vi "GetDisplayClick.vi"(0 "Display REFs In":refnum<vi>[](array[refnum]), 11 "Calling VI REF":refnum<vi>) -> (8 "Display Index":i32)   [LabVIEW 2014]
uses:
  <vilib>/Utility/cursorutil.llb/Set Cursor (Icon Pict).vi
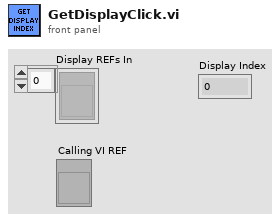
[diagram p1: front panel]
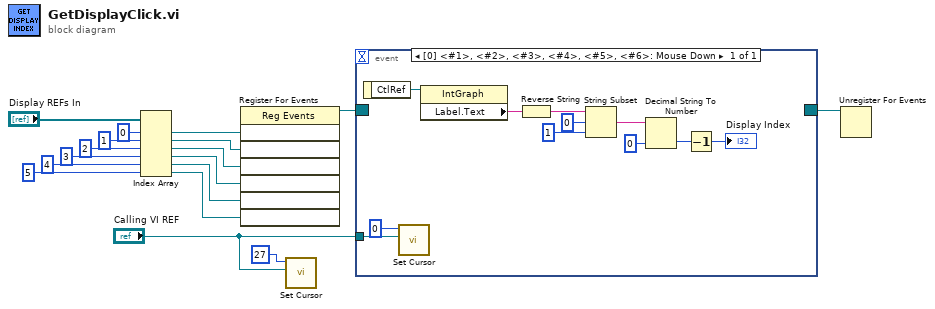
[diagram p0: block diagram]
diagram:
  n1 = Index Array(array="Display REFs In", index #1=0 ("index"), index #2=1 ("index"), index #3=2 ("index"), index #4=3 ("index"), index #5=4 ("index"), index #6=5 ("index")) -> (element #1=w4:refnum<vi>, element #2=w7:refnum<vi>, element #3=w8:refnum<vi>, element #4=w9:refnum<vi>, element #5=w10:refnum<vi>, element #6=w11:refnum<vi>)
  n2 = register-events(w4, w7, w8, w9, w10, w11) -> (reference out=w6:refnum<event-registration>)  [unwired: 2 in, 1 out]
  n3 = call-poly <vilib>:"Set Cursor.vi"("VI reference (current VI)"="Calling VI REF", "icon"=u16 27) -> ()  [unwired: 8 in, 2 out]
  n4 = event shown="[0] <#1>, <#2>, <#3>, <#4>, <#5>, <#6>: Mouse Down" {
    selector: w6 -> [_]
    dyn-events: [_] -> w5
    timeout: _ -> [_]
    tunnel: "Calling VI REF" -> [w27]
    event Mouse Down {
      n5 = event-data() -> ("CtlRef"=w26:refnum<vi>)  [unwired: 1 in]
      n6 = call-poly <vilib>:"Set Cursor.vi"("VI reference (current VI)"=w27, "icon"=u16 0) -> ()  [unwired: 8 in, 2 out]
      n7 = property class="IntGraph"(reference=w26) -> ("Label.Text"=w25:string)  [unwired: 1 in, 2 out]
      n8 = Reverse String(1:w25) -> (0:w24:string)
      n9 = String Subset(string=w24, offset (0)=0, length (rest)=1 ("length (rest)")) -> (substring=w21:string)
      n10 = Decimal String To Number(string=w21, default (0L)=0 ("default (0 I32)")) -> (number=w19:i32)  [unwired: 1 in, 1 out]
      n11 = Decrement(x=w19) -> (x-1=→"Display Index":i32)
    }
  }
  n12 = Unregister For Events(event registration refnum=w5) -> ()  [unwired: 1 in, 1 out]
